vi "testGUI.vi"() -> ()   [LabVIEW 2020]
panel:
  out "?":dbl
  out "4":bool
  out "?":dbl
  out "3":bool
  out "?":dbl
  out "2":bool
  out "?":dbl
  out "1":bool
  out "Right Side\nLens":dbl
  out "Right Front \nLens":dbl
  out "Left Front\nLens":dbl
  in  "ms":u32
  out "Left Side \nLens":dbl
  # "Freq (ms)"
  # "Voltage"
  # "Current"
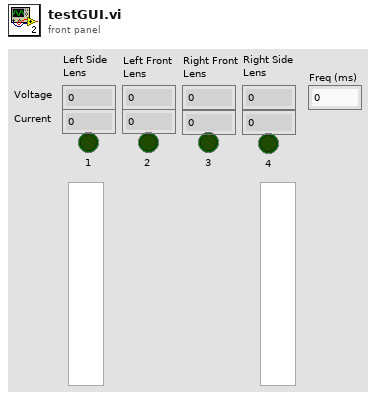
[diagram p1: front panel]
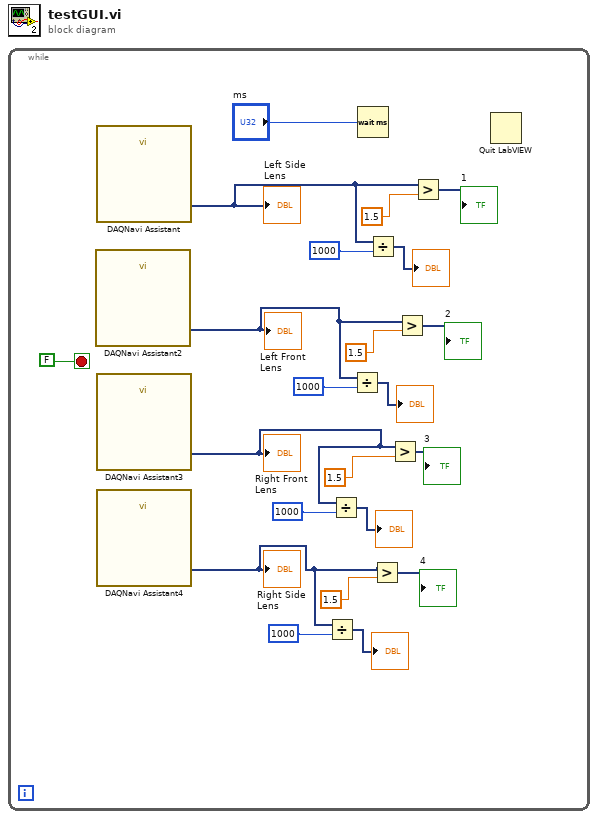
[diagram p0: block diagram]
diagram:
  n1 = while {
    stop <- FALSE ("stop") stop-if-true
    n2 = call "DAQNavi Assistant2"() -> ("data out(DDT)"=w12:dynamicdata)  [unwired: 26 in, 1 out]
    "Left Front\nLens" <- w12
    n3 = call "DAQNavi Assistant"() -> ("data out(DDT)"=w19:dynamicdata)  [unwired: 26 in, 1 out]
    "Left Side \nLens" <- w19
    n4 = call "DAQNavi Assistant3"() -> ("data out(DDT)"=w7:dynamicdata)  [unwired: 26 in, 1 out]
    "Right Front \nLens" <- w7
    n5 = call "DAQNavi Assistant4"() -> ("data out(DDT)"=w2:dynamicdata)  [unwired: 26 in, 1 out]
    "Right Side\nLens" <- w2
    n6 = Divide(x=w2, y=1000) -> (x/y=→"?":dynamicdata)
    n7 = Divide(x=w7, y=1000) -> (x/y=→"?":dynamicdata)
    n8 = Divide(x=w12, y=1000) -> (x/y=→"?":dynamicdata)
    n9 = Wait (ms)(milliseconds to wait="ms") -> ()  [unwired: 1 out]
    n10 = Divide(x=w19, y=1000) -> (x/y=→"?":dynamicdata)
    n11 = Greater?(x=w2, y=1.5) -> (0:→"4":dynamicdata)
    n12 = Greater?(x=w7, y=1.5) -> (0:→"3":dynamicdata)
    n13 = Greater?(x=w12, y=1.5) -> (0:→"2":dynamicdata)
    n14 = Greater?(x=w19, y=1.5) -> (0:→"1":dynamicdata)
    n15 = Quit LabVIEW() -> ()  [unwired: 1 in]
  }
